vi "Get All Vacuum.vi"(8 "error in":errorcluster, 11 "Gantry Class in":refnum<class "Gantry Class.lvclass">) -> (0 "error out":errorcluster, 2 "Channel Array":bool[](array[boolean]), 3 "Gantry Class out":refnum<class "Gantry Class.lvclass">)   [LabVIEW 2011]
uses:
  Gantry Class/Gantry Class.lvclass
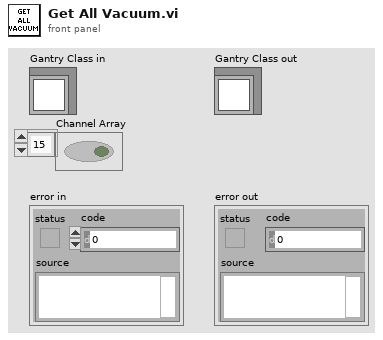
[diagram p1: front panel]
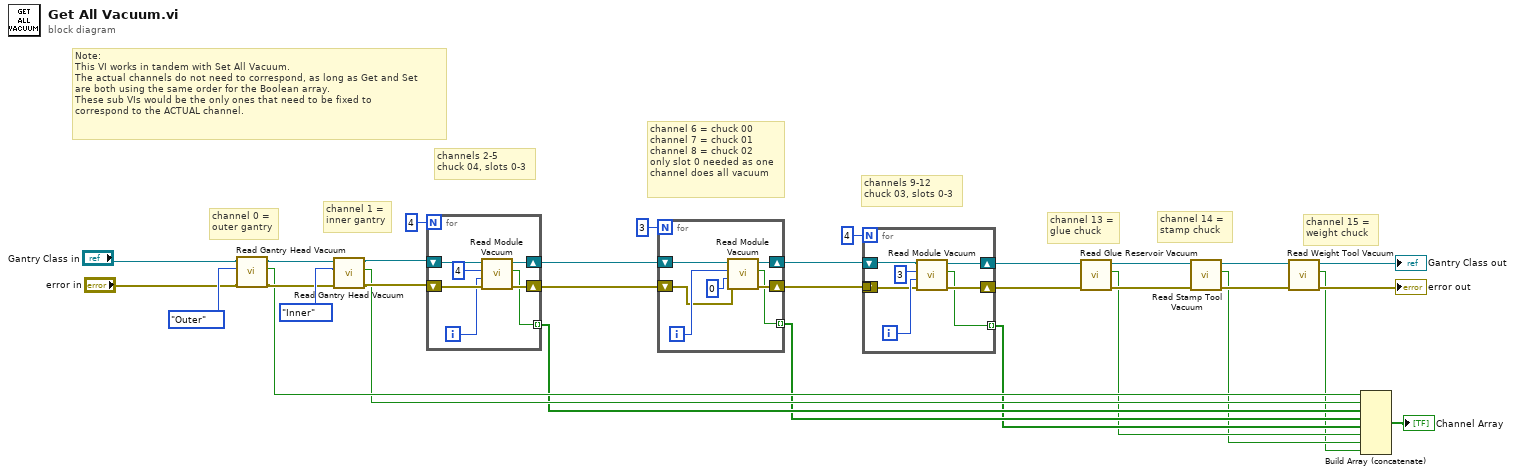
[diagram p0: block diagram]
diagram:
  # "Note:\nThis VI works in tandem with Set All Vacuum.\nThe actual channels do not need to correspond, as long as Get and Set\nare both using the same order for the Boolean array.\nThese sub VIs would be the only ones that need to be fixed to\ncorrespond to the ACTUAL channel."
  # "channel 15 =\nweight chuck"
  # "channel 14 = \nstamp chuck"
  # "channel 13 =\nglue chuck"
  # "channels 9-12\nchuck 03, slots 0-3"
  # "channel 6 = chuck 00\nchannel 7 = chuck 01\nchannel 8 = chuck 02\nonly slot 0 needed as one\nchannel does all vacuum"
  # "channels 2-5\nchuck 04, slots 0-3"
  # "channel 1 =\ninner gantry"
  # "channel 0 =\nouter gantry"
  n1 = call-dynamic "Read Gantry Head Vacuum.vi"("error in"="error in", "Inner/Outer"=enum16{"Outer", "Inner"}."Outer", "Gantry in"="Gantry Class in") -> ("error out"=w16:errorcluster, "On/Off"=w11:bool, "Gantry out"=w17:refnum<class "Gantry Class.lvclass">)  [unwired: 6 in]
  n2 = call-dynamic "Read Gantry Head Vacuum.vi"("error in"=w16, "Inner/Outer"=enum16{"Outer", "Inner"}."Inner", "Gantry in"=w17) -> ("error out"=w19:errorcluster, "On/Off"=w10:bool, "Gantry out"=w20:refnum<class "Gantry Class.lvclass">)  [unwired: 6 in]
  n3 = for {
    N: 4 -> [_]
    shift-right: [w39] -> w32
    shift-left: w20 -> [w34]
    shift-right: [w38] -> w31
    shift-left: w19 -> [w37]
    tunnel: [w33] -> w9 mode=indexing
    i -> [w35]
    n4 = call-dynamic "Read Module Vacuum.vi"("error in"=w37, "Slot Number"=w35, "Chuck Number"=4, "Gantry in"=w34) -> ("error out"=w38:errorcluster, "On/Off"=w33:bool, "Gantry out"=w39:refnum<class "Gantry Class.lvclass">)  [unwired: 5 in]
  }
  n5 = for {
    N: 3 -> [_]
    shift-right: [w46] -> w30
    shift-left: w32 -> [w41]
    shift-right: [w45] -> w29
    shift-left: w31 -> [w40]
    tunnel: [w44] -> w8 mode=indexing
    i -> [w42]
    n6 = call-dynamic "Read Module Vacuum.vi"("error in"=w40, "Slot Number"=0, "Chuck Number"=w42, "Gantry in"=w41) -> ("error out"=w45:errorcluster, "On/Off"=w44:bool, "Gantry out"=w46:refnum<class "Gantry Class.lvclass">)  [unwired: 5 in]
  }
  n7 = for {
    N: 4 -> [_]
    tunnel: w29 -> [_]
    shift-right: [w53] -> w22
    shift-left: w30 -> [w52]
    shift-right: [w48] -> w21
    shift-left: _ -> [w49]
    tunnel: [w47] -> w7 mode=indexing
    i -> [w50]
    n8 = call-dynamic "Read Module Vacuum.vi"("error in"=w49, "Slot Number"=w50, "Chuck Number"=3, "Gantry in"=w52) -> ("error out"=w48:errorcluster, "On/Off"=w47:bool, "Gantry out"=w53:refnum<class "Gantry Class.lvclass">)  [unwired: 5 in]
  }
  n9 = call-dynamic "Read Glue Reservoir Vacuum.vi"("error in"=w21, "Gantry in"=w22) -> ("error out"=w23:errorcluster, "On/Off"=w6:bool, "Gantry out"=w24:refnum<class "Gantry Class.lvclass">)  [unwired: 7 in]
  n10 = call-dynamic "Read Stamp Tool Vacuum.vi"("error in"=w23, "Gantry in"=w24) -> ("error out"=w25:errorcluster, "On/Off"=w5:bool, "Gantry out"=w26:refnum<class "Gantry Class.lvclass">)  [unwired: 7 in]
  n11 = call-dynamic "Read Weight Tool Vacuum.vi"("error in"=w25, "Gantry in"=w26) -> ("error out"=→"error out":errorcluster, "On/Off"=w4:bool, "Gantry out"=→"Gantry Class out":refnum<class "Gantry Class.lvclass">)  [unwired: 7 in]
  n12 = Build Array (concatenate)(w11, w10, w9, w8, w7, w6, w5, w4) -> (→"Channel Array":bool[])
